vi "ExtractDataAndHeader.vi"(9 "data array":dbl[][](array[numeric]), 10 "header array":cluster{"Enum":T1, "variable name":string}[](array[cluster]), 11 "Enum":T1) -> (2 "data sub array":dbl[][](array[numeric]), 3 "header subarray":cluster{"Enum":T1, "variable name":string}[](array[cluster]))   [LabVIEW 2018, in "MasterProgramSupportFunctions.lvlib"]
uses:
  MasterProgramSupportFunctions.lvlib
  VI_tags.ctl
panel:
  in  "array stop":i32
  in  "array start":i32
  in  "Array":string[](array[string])
  in  "intput array":dbl[][](array[numeric])
  out "output header":string
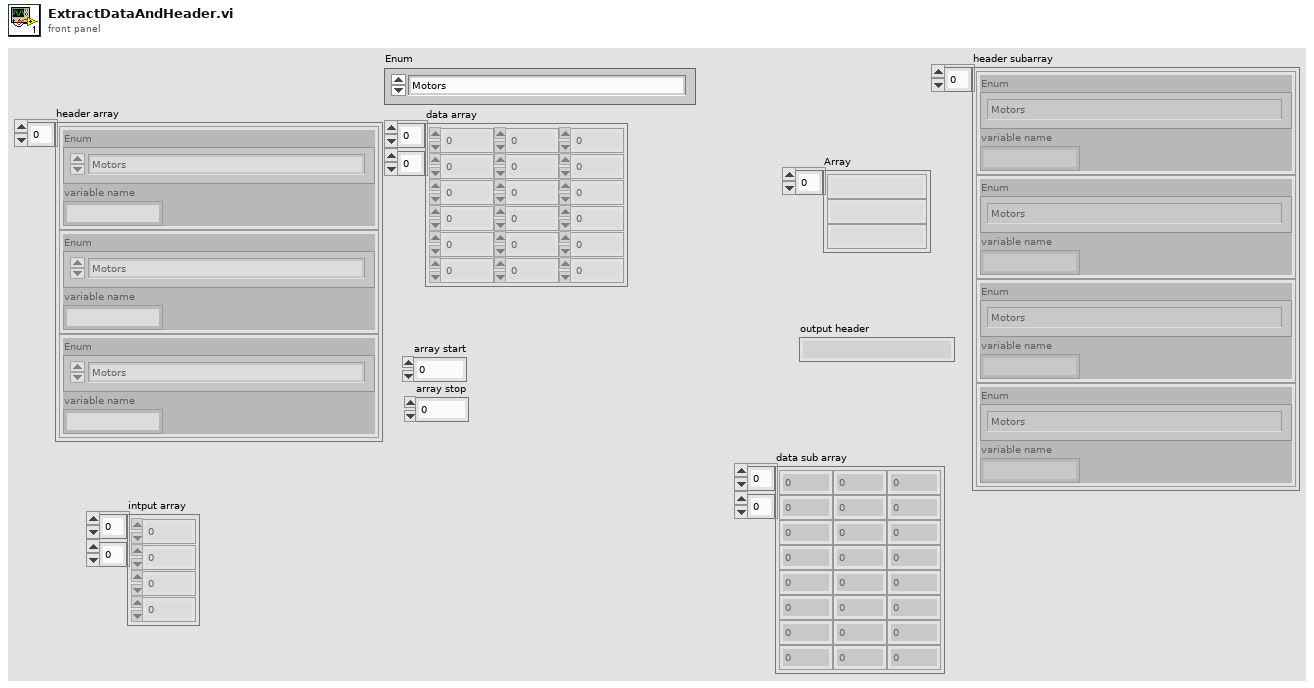
[diagram p1: front panel]
types:
  T1 = typedef "MasterProgramSupportFunctions.lvlib/VI_tags.ctl" = enum16{"Motors", "Gage", "Tektro3107", "XimeaMainCamera", "ContinuousMainScan"}
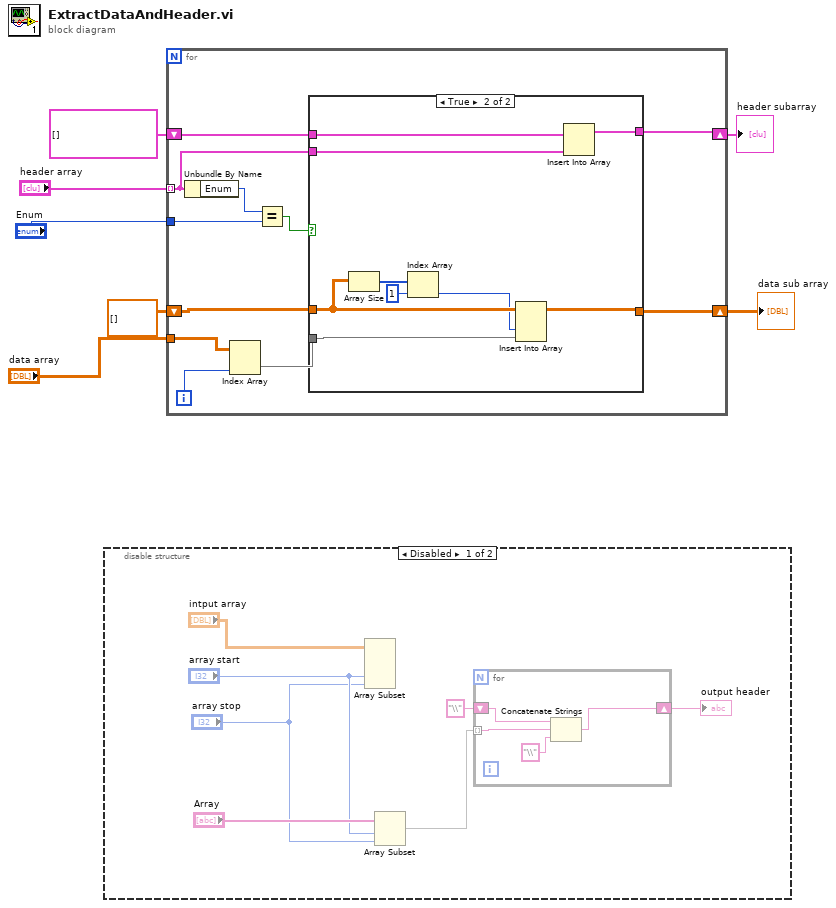
[diagram p0: block diagram]
diagram:
  n1 = disable-structure shown="Disabled" {
    frame Disabled {
      n2 = Array Subset(array="intput array", index (col)="array start", length (col)="array stop") -> (w11:dbl[][])  [unwired: 2 in]
      n3 = Array Subset(array="Array", index="array start", length="array stop") -> (w10:string[])
      n4 = for {
        shift-right: [w19] -> w15
        shift-left: "\\" -> [w18]
        tunnel: w10 -> [w16] mode=indexing
        n5 = Concatenate Strings(w18, w16, "\\" ("string")) -> (w19:string)
      }
      "output header" <- w15
    }
    frame Enabled {
    }
  }
  n6 = for {
    tunnel: "header array" -> [w27] mode=indexing
    tunnel: "Enum" -> [w28]
    shift-right: [w26] -> w4
    shift-left: cluster{"Enum":T1, "variable name":string}[] [] -> [w25]
    tunnel: "data array" -> [w22]
    shift-right: [w24] -> w1
    shift-left: dbl[][] [] -> [w23]
    i -> [w20]
    n7 = Unbundle By Name(w27) -> ("Enum"=w29:T1)
    n8 = Index Array(array=w22, index (col)=w20) -> (element=w21:dbl[])  [unwired: 1 in]
    n9 = Equal?(x=w29, y=w28) -> (x = y?=w30:bool)
    n10 = case shown="True" w30 {
      tunnel: w27 -> [_ w41]
      tunnel: [w32 w40] -> w26
      tunnel: w25 -> [w32 w39]
      tunnel: [w31 w38] -> w24
      tunnel: w23 -> [w31 w36]
      tunnel: w21 -> [_ w37]
      frame False {
      }
      frame True {
        n11 = Array Size(array=w36) -> (size(s)=w35:i32[])
        n12 = Index Array(array=w35, index=1) -> (element=w33:i32)
        n13 = Insert Into Array "Insert Into Array"(array=w36, index (col)=w33, new element=w37) -> (w38:dbl[][])  [unwired: 1 in]
        n14 = Insert Into Array(array=w39, new element=w41) -> (w40:cluster{"Enum":T1, "variable name":string}[])  [unwired: 1 in]
      }
    }
  }
  "header subarray" <- w4
  "data sub array" <- w1
